vi "PasaUnitatsString_a_ListBox.vi"(1 "UnitatsC2":string) -> (0 "Value":i32[](array[numeric]))   [LabVIEW 2017]
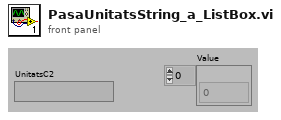
[diagram p1: front panel]
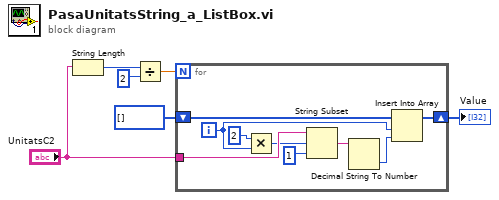
[diagram p0: block diagram]
diagram:
  n1 = String Length(string="UnitatsC2") -> (length=w1:i32)
  n2 = Divide(x=w1, y=2) -> (x/y=w3:dbl)
  n3 = for {
    N: w3 -> [_]
    tunnel: "UnitatsC2" -> [w15]
    shift-right: [w7] -> w6
    shift-left: i32[] [] ("Value") -> [w10]
    i -> [w9]
    n4 = Multiply(x=2, y=w9) -> (x*y=w12:i32)
    n5 = String Subset(string=w15, offset (0)=w12, length (rest)=1 ("length (rest)")) -> (substring=w11:string)
    n6 = Decimal String To Number(string=w11) -> (number=w8:i32)  [unwired: 2 in, 1 out]
    n7 = Insert Into Array(array=w10, index=w9, new element=w8) -> (w7:i32[])
  }
  "Value" <- w6
